vi "test Loopback Read Write RTs and BC.vi"(8 "error in":errorcluster, 11 "Loopback in":refnum<class "Loopback.lvclass">) -> (0 "error out":errorcluster, 3 "Loopback out":refnum<class "Loopback.lvclass">)   [LabVIEW 2020, in "Loopback.lvclass"]
uses:
  Loopback.lvclass
  <vilib>/NI/VeriStand Custom Device Testing Tools/VeriStandTestUtilities/VeriStandTestUtilities.lvlib
  <vilib>/numeric/Random Number (Range) U64.vi
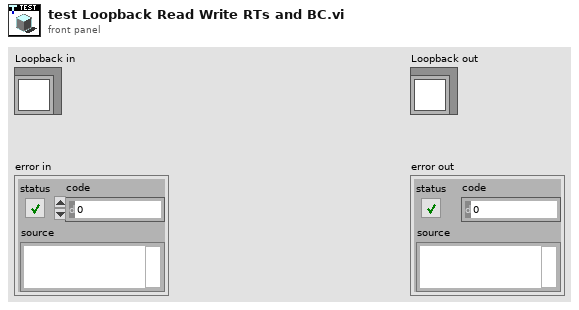
[diagram p1: front panel]
types:
  T1 = typedef "NI_VS Workspace ExecutionAPI.lvlib/WorkspaceAPI.ctl" = refnum<k24>
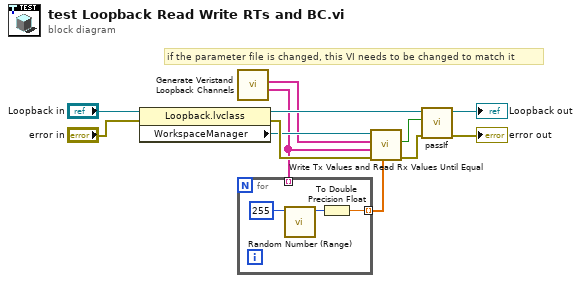
[diagram p0: block diagram]
diagram:
  # "if the parameter file is changed, this VI needs to be changed to match it"
  n1 = property class="Loopback.lvclass"(reference="Loopback in", error in="error in") -> (reference out=w5:refnum<class "Loopback.lvclass">, error out=w6:errorcluster, "WorkspaceManager"=w4:T1)
  n2 = call "Generate Veristand Loopback Channels.vi"() -> ("Rx Aliases"=w2:string[], "Tx Aliases"=w3:string[])  [unwired: 10 in]
  n3 = for {
    tunnel: [w13] -> w1 mode=indexing
    tunnel: w2 -> [_] mode=indexing
    n4 = call-poly <vilib>:"Random Number (Range).vi"("upper bound (100)"=u64 255) -> ("number"=w15:u64)  [unwired: 10 in]
    n5 = To Double Precision Float(number=w15) -> (double precision float=w13:dbl)
  }
  n6 = call <vilib>:"Write Tx Values and Read Rx Values Until Equal.vi"("Tx values"=w1, "error in"=w6, "Rx aliases"=w2, "Tx aliases"=w3, "workspace manager in"=w4) -> ("error out"=w11:errorcluster, "values equal"=w12:bool)  [unwired: 4 in, 1 out]
  n7 = call-dynamic "passIf.vi"("error in (no error)"=w11, "pass"=w12, "TestCase in"=w5) -> ("error out"=→"error out":errorcluster, "TestCase out"=→"Loopback out":refnum<class "Loopback.lvclass">)  [unwired: 7 in]
